vi "Cleanup.vi"(8 "error in (no error)":errorcluster, 11 "LV Chat Server in":refnum<class "LV Chat Server.lvclass">) -> (0 "error out":errorcluster)   [LabVIEW 2020, in "LV Chat Server.lvclass"]
uses:
  LV Chat Server.lvclass
  LV Chat Server.lvclass/LV Chat Server.ctl
  <vilib>/IlluminatedG/lv-msg-simple/Stream-Simple-Msg/Manager/Manager.lvclass
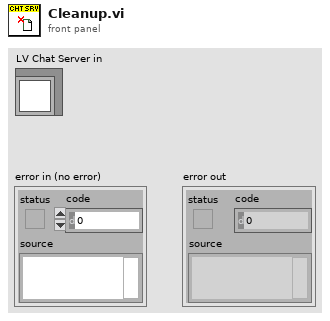
[diagram p1: front panel]
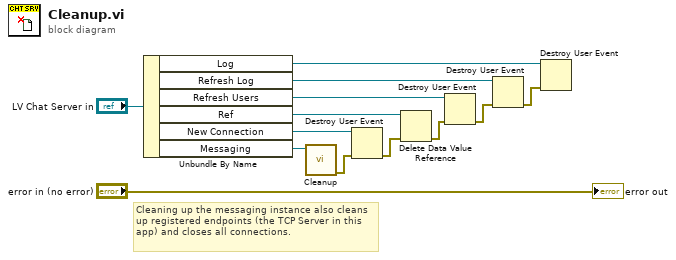
[diagram p0: block diagram]
diagram:
  # "Cleaning up the messaging instance also cleans up registered endpoints (the TCP Server in this app) and closes all connections."
  n1 = Unbundle By Name("LV Chat Server in") -> ("Log"=w2:refnum<user-event>, "Refresh Log"=w4:refnum<user-event>, "Refresh Users"=w6:refnum<user-event>, "Ref"=w10:refnum<data-value>, "New Connection"=w11:refnum<user-event>, "Messaging"=w8:refnum<class "Manager.lvclass">)
  n2 = call <vilib>:"Cleanup.vi"("Manager in"=w8) -> ("error out"=w7:errorcluster)  [unwired: 10 in]
  n3 = Destroy User Event(user event=w11, error in=w7) -> (error out=w9:errorcluster)
  n4 = Delete Data Value Reference(data value reference=w10, error in=w9) -> (error out=w5:errorcluster)  [unwired: 1 out]
  n5 = Destroy User Event(user event=w6, error in=w5) -> (error out=w3:errorcluster)
  n6 = Destroy User Event(user event=w4, error in=w3) -> (error out=w1:errorcluster)
  n7 = Destroy User Event(user event=w2, error in=w1) -> ()  [unwired: 1 out]
  "error out" <- "error in (no error)"
